vi "Shared Variable Client - Variable API.vi"() -> ()   [LabVIEW 2016]
doc: "This client VI connects to Shared Variable Server.vi by using the Shared Variable API to read the server variable values."
panel:
  in  "Stop":bool
  out "Monitor Value 1":dbl
  out "Monitor Value 2":dbl
  # "Overview: Demonstrates the use of the Shared Variable API functions to read shared variable data from a server VI.\nRequirements: Windows\nInstructions:\n1. Make sure Shared Variable Server.vi is already running.\n2. Run this VI. It will read the values of the server shared variables through the Shared Variable API.\n3. Click Stop to stop the VI."
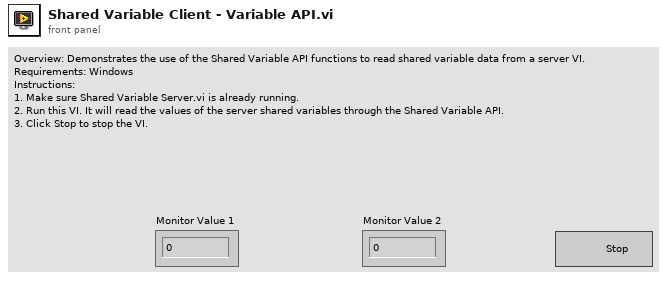
[diagram p1: front panel]
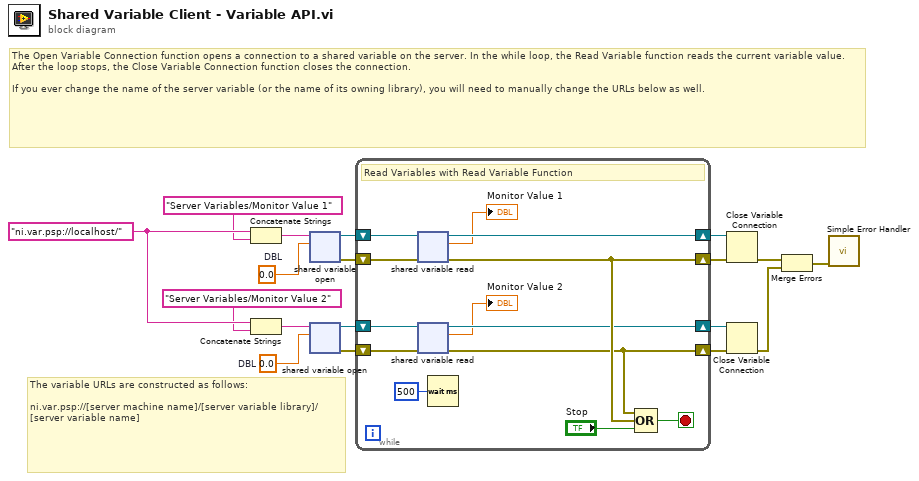
[diagram p0: block diagram]
diagram:
  w1 = 0.0  # DBL
  w2 = 0.0  # DBL
  w18 = "ni.var.psp://localhost/" ("string")
  # "The Open Variable Connection function opens a connection to a shared variable on the server. In the while loop, the Read Variable function reads the current variable value. After the loop stops, the Close Variable Connection function closes the connection.\n\nIf you ever change the name of the server variable (or the name of its owning library), you will need to manually change the URLs below as well."
  # "The variable URLs are constructed as follows:\n\nni.var.psp://[server machine name]/[server variable library]/[server variable name]"
  n1 = Concatenate Strings(w18, "Server Variables/Monitor Value 1") -> (w3:string)
  n2 = Concatenate Strings(w18, "Server Variables/Monitor Value 2") -> (w13:string)
  n3 = shared-variable-open(w3, w2) -> (w8:refnum<k21>, w7:errorcluster)  [unwired: 2 in]
  n4 = shared-variable-open(w13, w1) -> (w9:refnum<k21>, w10:errorcluster)  [unwired: 2 in]
  n5 = while {
    shift-right: [w30] -> w6
    shift-left: w8 -> [w29]
    shift-right: [w27] -> w4
    shift-left: w7 -> [w28]
    shift-right: [w21] -> w11
    shift-left: w9 -> [w22]
    shift-right: [w19] -> w12
    shift-left: w10 -> [w23]
    stop <- w26 stop-if-true
    # "Read Variables with Read Variable Function"
    n6 = shared-variable-read(w29, w28) -> (w30:refnum<k21>, w27:errorcluster, →"Monitor Value 1":dbl)  [unwired: 1 out]
    n7 = shared-variable-read(w22, w23) -> (w21:refnum<k21>, w19:errorcluster, →"Monitor Value 2":dbl)  [unwired: 1 out]
    n8 = Wait (ms)(milliseconds to wait=u32 500 ("millisecond multiple")) -> ()  [unwired: 1 out]
    n9 = Compound Arithmetic op=OR(w19, w27, "Stop") -> (w26:bool)
  }
  n10 = Close Variable Connection(8:w4, 11:w6) -> (0:w5:errorcluster)
  n11 = Close Variable Connection(8:w12, 11:w11) -> (0:w16:errorcluster)
  n12 = Merge Errors(w5, w16) -> (w15:errorcluster)
  n13 = call <vilib>:"Simple Error Handler.vi"("error in (no error)"=w15) -> ()  [unwired: 4 in, 5 out]
